vi "FeedbackDecode_ConvertDates.vi"(1 "Dates":string[](array[string])=["10/14/2011\u0000\u0000\u0000\u0000\u0000\u0000\u0000\u0000\u0000\u0000\u0000\u0000", "10/14/2011 11:14:43 PM", "10/14/2011 3:56:30 PM\u0000", "10/14/2011 4:18:24 PM\u0000", "10/15/2011\u0000\u0000\u0000\u0000\u0000\u0000\u0000\u0000\u0000\u0000\u0000\u0000", "10/15/2011 7:54:35 AM\u0000", "10/16/2011\u0000\u0000\u0000\u0000\u0000\u0000\u0000\u0000\u0000\u0000\u0000\u0000"]) -> (0 "ConvertedDates":string[](array[string]))   [LabVIEW 2020]
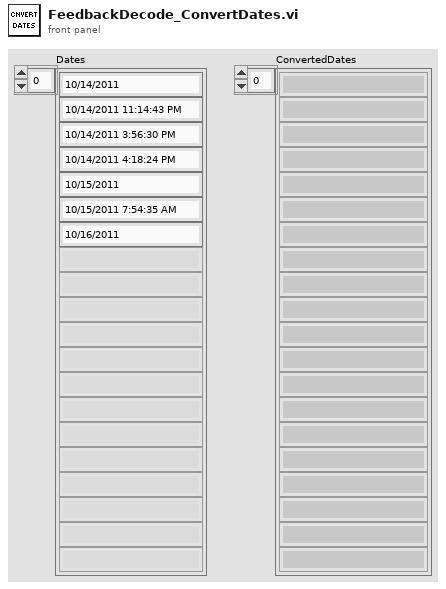
[diagram p1: front panel]
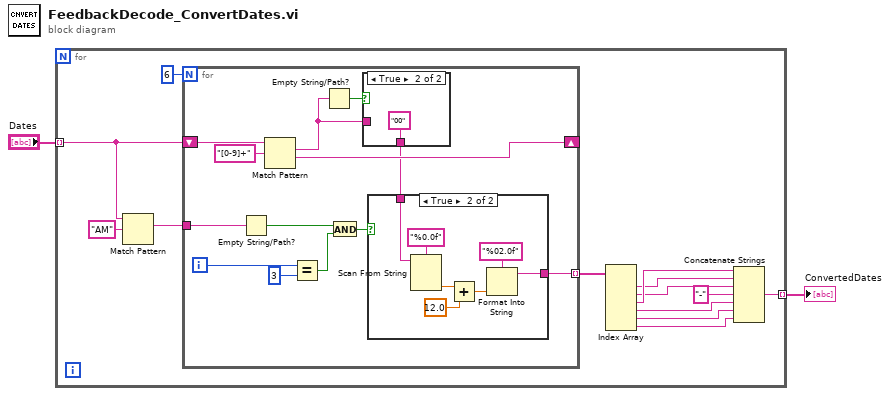
[diagram p0: block diagram]
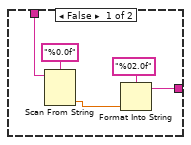
[diagram p3: hidden frame]
diagram:
  n1 = for {
    tunnel: "Dates" -> [w13] mode=indexing
    tunnel: [w5] -> w1 mode=indexing
    n2 = Match Pattern(string=w13, regular expression="AM") -> (match substring=w12:string)  [unwired: 1 in, 3 out]
    n3 = for {
      N: 6 -> [_]
      shift-right: [w27] -> _
      shift-left: w13 -> [w26]
      tunnel: w12 -> [w22]
      tunnel: [w19] -> w11 mode=indexing
      i -> [w25]
      n4 = Empty String/Path?(string/path=w22) -> (empty?=w21:bool)
      n5 = Match Pattern(string=w26, regular expression="[0-9]+") -> (match substring=w17:string, after substring=w27:string)  [unwired: 1 in, 2 out]
      n6 = Equal?(x=w25, y=3) -> (x = y?=w23:bool)
      n7 = Empty String/Path?(string/path=w17) -> (empty?=w18:bool)
      n8 = And(x=w21, y=w23) -> (x .and. y?=w20:bool)
      n9 = case shown="True" w18 {
        tunnel: w17 -> [w29 _]
        tunnel: [w29 "00"] -> w16
        frame False {
        }
        frame True {
        }
      }
      n10 = case shown="True" w20 {
        tunnel: w16 -> [w33 w42]
        tunnel: [w31 w37] -> w19
        frame False {
          n11 = Scan From String(format string="%0.0f", input string=w33) -> (output 1=w32:dbl)  [unwired: 3 in, 3 out]
          n12 = Format Into String(format string="%02.0f", w32) -> (resulting string=w31:string)  [unwired: 2 in, 1 out]
        }
        frame True {
          n13 = Scan From String(format string="%0.0f", input string=w42) -> (output 1=w41:dbl)  [unwired: 3 in, 3 out]
          n14 = Add(x=w41, y=12.0) -> (x+y=w39:dbl)
          n15 = Format Into String(format string="%02.0f", w39) -> (resulting string=w37:string)  [unwired: 2 in, 1 out]
        }
      }
    }
    n16 = Index Array(array=w11) -> (element #1=w4:string, element #2=w3:string, element #3=w10:string, element #4=w8:string, element #5=w7:string, element #6=w6:string)  [unwired: 6 in]
    n17 = Concatenate Strings(w10, w4, w3, "-" ("string"), w8, w7, w6) -> (w5:string)
  }
  "ConvertedDates" <- w1
